vi "sterowaniePlatforma.vi"() -> ()   [LabVIEW 2017]
panel:
  out "data out":string
  in  "readTCP":bool
  in  "stop":bool
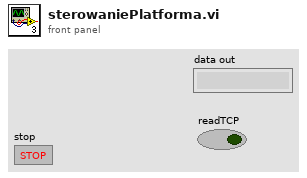
[diagram p1: front panel]
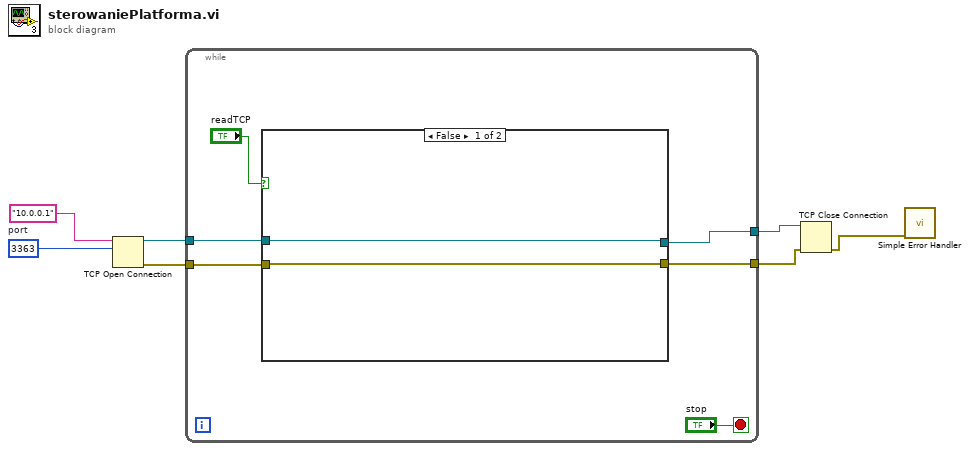
[diagram p0: block diagram]
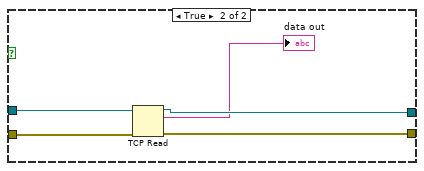
[diagram p2: hidden frame]
diagram:
  w7 = u16 3363  # port
  n1 = TCP Open Connection(address="10.0.0.1", remote port or service name=w7) -> (connection ID=w6:refnum<k5>, error out=w4:errorcluster)  [unwired: 3 in]
  n2 = while {
    tunnel: w6 -> [w11]
    tunnel: [w10] -> w5
    tunnel: w4 -> [w9]
    tunnel: [w8] -> w3
    stop <- "stop" stop-if-true
    n3 = case shown="False" "readTCP" {
      tunnel: w11 -> [w14 w20]
      tunnel: [w14 w19] -> w10
      tunnel: w9 -> [w15 w18]
      tunnel: [w15 w17] -> w8
      frame False {
      }
      frame True {
        n4 = TCP Read(connection ID=w20, error in (no error)=w18) -> (connection ID out=w19:refnum<k5>, data out=→"data out":string, error out=w17:errorcluster)  [unwired: 3 in]
      }
    }
  }
  n5 = TCP Close Connection(connection ID=w5, error in (no error)=w3) -> (error out=w2:errorcluster)  [unwired: 1 in, 1 out]
  n6 = call <vilib>:"Simple Error Handler.vi"("error in (no error)"=w2) -> ()  [unwired: 4 in, 5 out]
